vi "GetText.vi"(0 "reference in":refnum<class "Text.lvclass">, 5 "error in (no error)":errorcluster) -> (14 "reference out":refnum<class "Text.lvclass">, 16 "Text":string, 19 "error out":errorcluster)   [LabVIEW 2014, in "FrontPanelPublisher.lvlib" / "Text.lvclass"]
uses:
  Text.lvclass
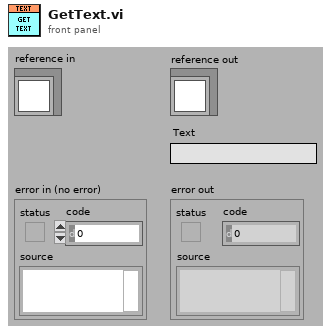
[diagram p1: front panel]
types:
  T1 = typedef "FrontPanelPublisher.lvlib/Text.lvclass/Attributes.ctl" = cluster{"Text":string, "Font":string, "Font Size":u32, "Visible":bool}
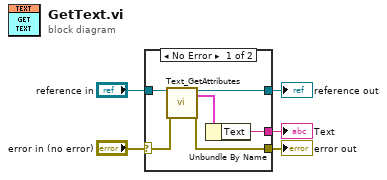
[diagram p0: block diagram]
diagram:
  n1 = case shown="No Error" "error in (no error)" {
    selector: "error in (no error)" -> [w11 w13]
    tunnel: [w9 w13] -> w4
    tunnel: [w7 w12] -> w2
    tunnel: "reference in" -> [w8 w12]
    tunnel: [w6 _] -> w1
    frame No Error {
      n2 = call "Text_GetAttributes.vi"("reference in"=w8, "error in (no error)"=w11) -> ("reference out"=w7:refnum<class "Text.lvclass">, "Data"=w10:T1, "error out"=w9:errorcluster)  [unwired: 14 in, 1 out]
      n3 = Unbundle By Name(w10) -> ("Text"=w6:string)
    }
    frame Error {
    }
  }
  "error out" <- w4
  "reference out" <- w2
  "Text" <- w1
